vi "Destroy Image Window.vi"(8 "error in (no error)":errorcluster, 11 "Window Name":string) -> (0 "error out":errorcluster, 3 "Already Closed":bool)   [LabVIEW 2020, in "g_ar_toolkit.image.lvlib"]
uses:
  g_ar_toolkit.image.lvlib
  g_ar_toolkit.common/g_ar_toolkit.common.lvlib
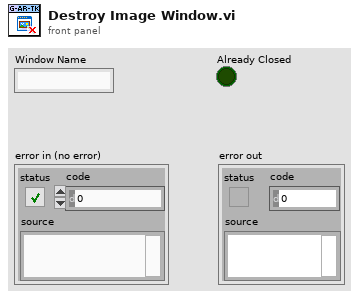
[diagram p1: front panel]
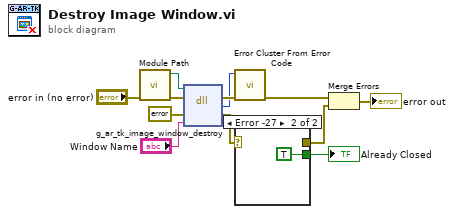
[diagram p0: block diagram]
diagram:
  n1 = call "Module Path.vi"("error in (no error)"="error in (no error)") -> ("error out"=w2:errorcluster, "Path"=w1:path)  [unwired: 9 in]
  n2 = dll-call lib="?" fn="g_ar_tk_image_window_destroy"(path in=w1, error in=w2, "error_cluster"=errorcluster {"status"=FALSE, "code"=0, "source"=""} ("error constant"), "window_name"="Window Name") -> (error out=w12:errorcluster, "MgErr"=w11:i32, "error_cluster"=w5:errorcluster)  [unwired: 2 in, 1 out]
  n3 = call <vilib>:"Error Cluster From Error Code.vi"("error in (no error)"=w12, "error code (0)"=w11) -> ("error out"=w10:errorcluster)  [unwired: 7 in]
  n4 = case shown="Error -27" w5 {
    selector: w5 -> [w13 _]
    tunnel: [w13 _] -> w4
    tunnel: [_ TRUE] -> w3
    frame #0 {
    }
    frame #1 {
    }
  }
  "Already Closed" <- w3
  n5 = Merge Errors(w10, w4) -> (→"error out":errorcluster)
